vi "Run Bfr Tx - FIFO Port.vi"(7 "Buffer in":u64, 8 "error in (no error)":errorcluster, 11 "Offset in":u64) -> (0 "error out":errorcluster, 1 "Dest Port":u16, 3 "Offset out":u64, 5 "Buffer out":u64)   [LabVIEW 2019, in "UDP-Custom-Device Engine.lvlib"]
uses:
  UDP-Custom-Device Engine.lvlib
  <vilib>/NI VeriStand/VeriStand Data/Pointer Operations/Pointer.Read (U16).vi
  <vilib>/NI VeriStand/VeriStand Data/Pointer Operations/Pointer.In-Place Read (U16).vi
  <vilib>/NI VeriStand/VeriStand Data/VeriStand Data.lvlib
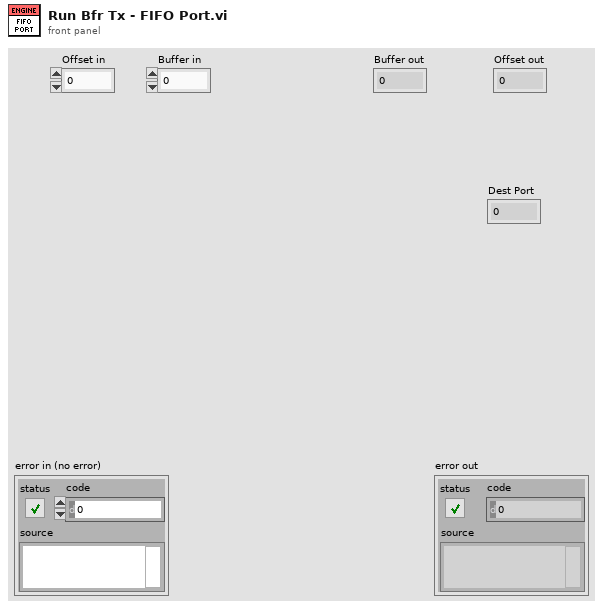
[diagram p1: front panel]
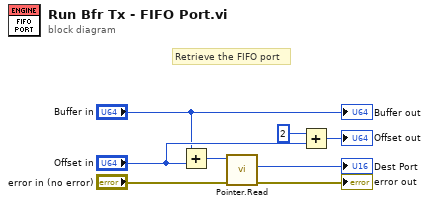
[diagram p0: block diagram]
diagram:
  # "Retrieve the FIFO port"
  n1 = Add(x="Buffer in", y="Offset in") -> (x+y=w4:u64)
  n2 = call-poly <vilib>:"Pointer.Read.vi"("error in (no error)"="error in (no error)", "pointer in"=w4) -> ("error out"=→"error out":errorcluster, "value"=→"Dest Port":u16)  [unwired: 7 in, 1 out]
  n3 = Add(x=u64 2, y="Offset in") -> (x+y=→"Offset out":u64)
  "Buffer out" <- "Buffer in"
